vi "Close_Top_Level_VIs.vi"(8 "error in (no error)":errorcluster, 10 "Top-Level VIs":refnum<vi>[](array[refnum]), 11 "AB_Build in":refnum<class "AB_Build.lvclass">) -> (0 "error out":errorcluster, 3 "AB_Build out":refnum<class "AB_Build.lvclass">)   [LabVIEW 2020, in "AB_Build.lvclass"]
uses:
  <vilib>/AppBuilder/AB_Classes/Build/AB_Build.lvclass
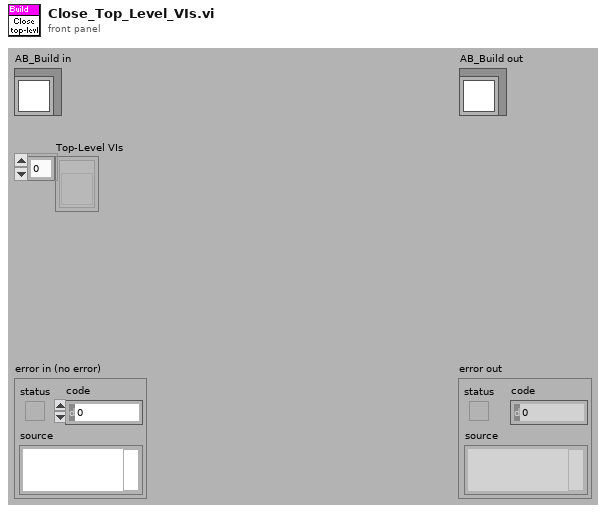
[diagram p1: front panel]
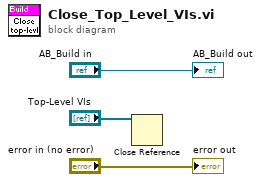
[diagram p0: block diagram]
diagram:
  n1 = Close Reference(reference="Top-Level VIs") -> ()  [unwired: 1 in, 1 out]
  "error out" <- "error in (no error)"
  "AB_Build out" <- "AB_Build in"
